vi "Initialize Tricon.vi"(8 "error IO":errorcluster, 11 "VISA resource name":refnum<visa-resource-name>="COM3") -> (0 "error out":errorcluster, 1 "Status Code":string, 2 "Connected":bool, 3 "VISA resource name Out":refnum<visa-resource-name>)   [LabVIEW 2018]
uses:
  Pump Address.ctl
panel:
  out "Value":dbl
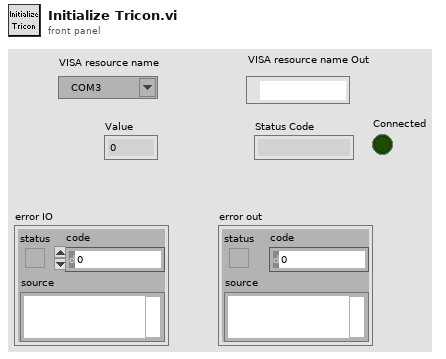
[diagram p1: front panel]
types:
  T1 = typedef "Pump Address.ctl" = enum16{"0", "1", "2", "3", "4", "5", "6", "7"}
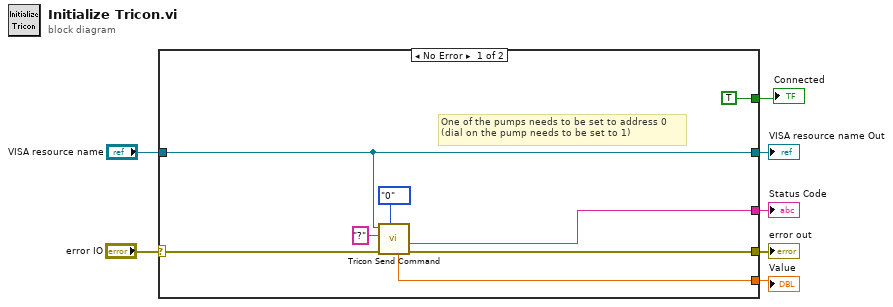
[diagram p0: block diagram]
diagram:
  n1 = case shown="No Error" "error IO" {
    selector: "error IO" -> [w14 w16]
    tunnel: [w13 w16] -> w7
    tunnel: "VISA resource name" -> [w12 _]
    tunnel: [w12 _] -> w4
    tunnel: [w10 _] -> w2
    tunnel: [w9 _] -> w3
    tunnel: [TRUE ("Connected") _] -> w1
    frame No Error {
      # "One of the pumps needs to be set to address 0\n(dial on the pump needs to be set to 1)"
      n2 = call "Tricon Send Command.vi"("Address"=Pump_Address."0" ("Pump Address"), "error in (no error)"=w14, "Command"="?", "VISA resource name in"=w12) -> ("error out"=w13:errorcluster, "Status Code"=w9:string, "Value"=w10:dbl)  [unwired: 3 in, 2 out]
    }
    frame Error {
    }
  }
  "error out" <- w7
  "VISA resource name Out" <- w4
  "Status Code" <- w3
  "Value" <- w2
  "Connected" <- w1
